vi "AlliGator Python Plugin Get Function Name.vi"(8 "Error In":errorcluster, 9 "Source":string, 11 "String in":string) -> (0 "Error Out":errorcluster, 1 "function_name":string, 2 "Is preceded by Separator":bool, 3 "String out":string)   [LabVIEW 2021, in "AlliGator Python Plugins.lvlib"]
doc: "Returns function name and whether the function should be preceded by a separator in the menu."
uses:
  AlliGator Python Plugins.lvlib
  <userlib>/_OpenG.lib/string/string.llb/openg_string.lvlib
panel:
  # "see the AlliGator License on the block diagram (Ctrl+E or Window:Show Block Diagram)"
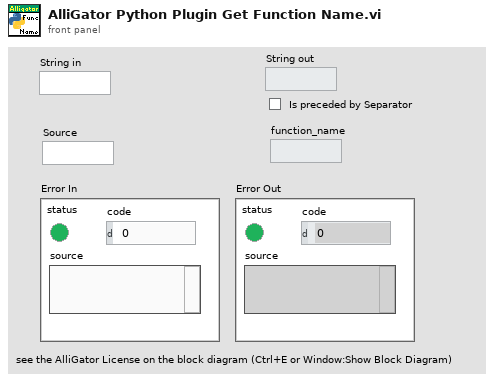
[diagram p1: front panel]
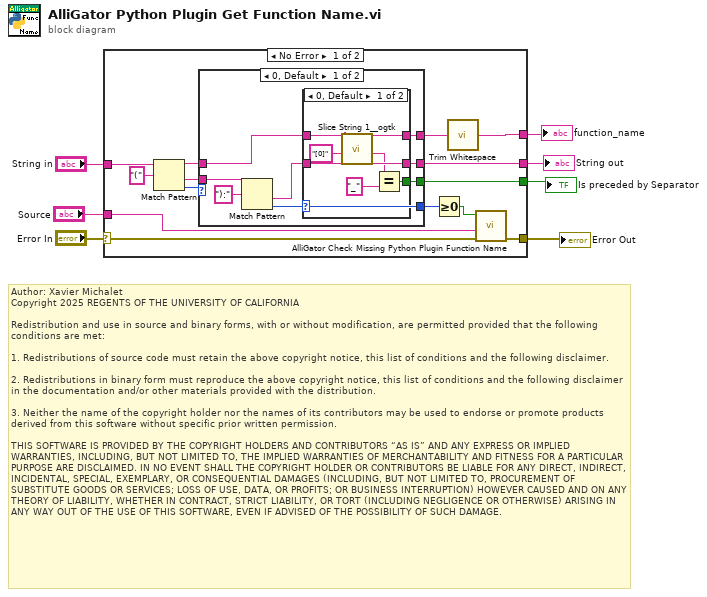
[diagram p0: block diagram]
diagram:
  # "Author: Xavier Michalet\nCopyright 2025 REGENTS OF THE UNIVERSITY OF CALIFORNIA\n\nRedistribution and use in source and binary forms, with or without modification, are permitted provided that the following conditions are met:\n\n1. Redistributions of source code must retain the above copyright notice, this list of conditions and the following disclaimer.\n\n2. Redistributions in binary form must reproduce the above copyright notice, this list of conditions and the following disclaimer in the documentation and/or other materials provided with the distribution.\n\n3. Neither the name of the copyright holder nor the names of its contributors may be used to endorse or promote products derived from this software without specific prior written permission.\n\nTHIS SOFTWARE IS PROVIDED BY THE COPYRIGHT HOLDERS AND CONTRIBUTORS “AS IS” AND ANY EXPRESS OR IMPLIED WARRANTIES, INCLUDING, BUT NOT LIMITED TO, THE IMPLIED WARRANTIES OF MERCHANTABILITY AND FITNESS FOR A PARTICULAR PURPOSE ARE DISCLAIMED. IN NO EVENT SHALL THE COPYRIGHT HOLDER OR CONTRIBUTORS BE LIABLE FOR ANY DIRECT, INDIRECT, INCIDENTAL, SPECIAL, EXEMPLARY, OR CONSEQUENTIAL DAMAGES (INCLUDING, BUT NOT LIMITED TO, PROCUREMENT OF SUBSTITUTE GOODS OR SERVICES; LOSS OF USE, DATA, OR PROFITS; OR BUSINESS INTERRUPTION) HOWEVER CAUSED AND ON ANY THEORY OF LIABILITY, WHETHER IN CONTRACT, STRICT LIABILITY, OR TORT (INCLUDING NEGLIGENCE OR OTHERWISE) ARISING IN ANY WAY OUT OF THE USE OF THIS SOFTWARE, EVEN IF ADVISED OF THE POSSIBILITY OF SUCH DAMAGE."
  n1 = case shown="No Error" "Error In" {
    selector: "Error In" -> [w14 w39]
    tunnel: [w21 w40] -> w7
    tunnel: "String in" -> [w19 w40]
    tunnel: [w8 _] -> w5
    tunnel: [w12 w39] -> w3
    tunnel: "Source" -> [w13 _]
    tunnel: [w9 _] -> w1
    frame No Error {
      n2 = Match Pattern(string=w19, regular expression="(") -> (before substring=w16:string, after substring=w20:string, offset past match=w17:i32)  [unwired: 1 in, 1 out]
      n3 = case shown="0, Default" w17 {
        selector: w17 -> [_ w37]
        tunnel: [w25 w38] -> w21
        tunnel: w20 -> [w28 _]
        tunnel: w16 -> [w26 w38]
        tunnel: [w24 _] -> w15
        tunnel: [w23 w37] -> w11
        tunnel: [w22 _] -> w9
        frame 0, Default {
          n4 = Match Pattern(string=w28, regular expression="):") -> (after substring=w27:string, offset past match=w23:i32)  [unwired: 1 in, 2 out]
          n5 = case shown="0, Default" w23 {
            tunnel: w27 -> [w35 _]
            tunnel: w26 -> [w34 w36]
            tunnel: [w35 w36] -> w25
            tunnel: [w34 _] -> w24
            tunnel: [w30 _] -> w22
            frame 0, Default {
              n6 = call <userlib>:"Slice String 1__ogtk.vi"("Subset (i:j)"="[0]", "String"=w34) -> ("Substring (String[i:j])"=w32:string)  [unwired: 7 in]
              n7 = Equal?(x=w32, y="_") -> (x = y?=w30:bool)
            }
            frame -1 {
            }
          }
        }
        frame -1 {
        }
      }
      n8 = Greater Or Equal To 0?(x=w11) -> (x >= 0?=w10:bool)
      n9 = call <vilib>:"Trim Whitespace.vi"("string"=w15) -> ("trimmed string"=w8:string)  [unwired: 1 in]
      n10 = call "AlliGator Check Missing Python Plugin Function Name.vi"("error in (no error)"=w14, "Source"=w13, "Function Name Found"=w10) -> ("error out"=w12:errorcluster)  [unwired: 8 in]
    }
    frame Error {
    }
  }
  "String out" <- w7
  "function_name" <- w5
  "Error Out" <- w3
  "Is preceded by Separator" <- w1
